vi "get desired keys.vi"(8 "error in":errorcluster, 11 "ScaleAndLimitModule configuration in":refnum<class "ScaleAndLimitModule configuration.lvclass">) -> (0 "error out":errorcluster, 2 "desired keys":string[](array[string]), 3 "ScaleAndLimitModule configuration out":refnum<class "ScaleAndLimitModule configuration.lvclass">)   [LabVIEW 2017, in "ScaleAndLimitModule configuration.lvclass"]
uses:
  ScaleAndLimitModule configuration.lvclass
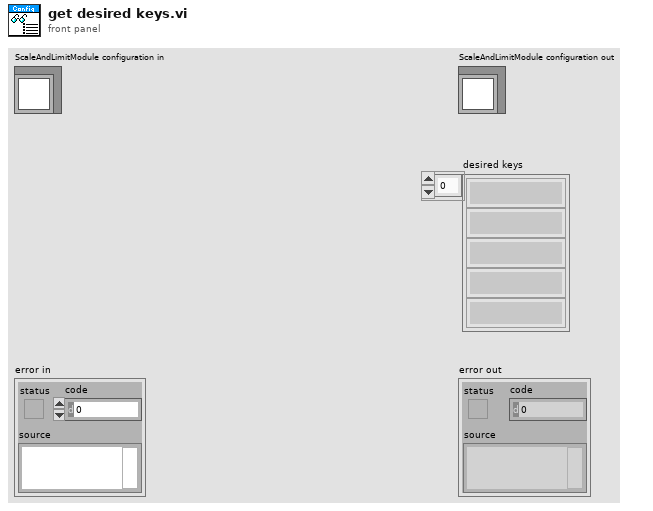
[diagram p1: front panel]
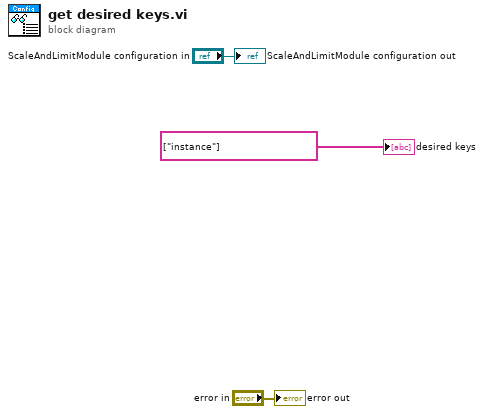
[diagram p0: block diagram]
diagram:
  "error out" <- "error in"
  "ScaleAndLimitModule configuration out" <- "ScaleAndLimitModule configuration in"
  "desired keys" <- string[] ["instance"] ("desired keys")
